vi "FindIP.vi"(2 "error in 2":errorcluster, 3 "String":string) -> (0 "error out":errorcluster, 1 "Numeric":u32)   [LabVIEW 2010]
uses:
  <vilib>/Utility/file.llb/Read From Spreadsheet File (string).vi
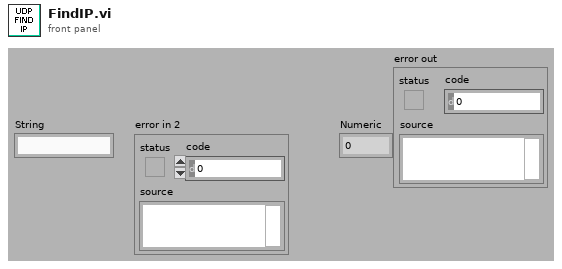
[diagram p1: front panel]
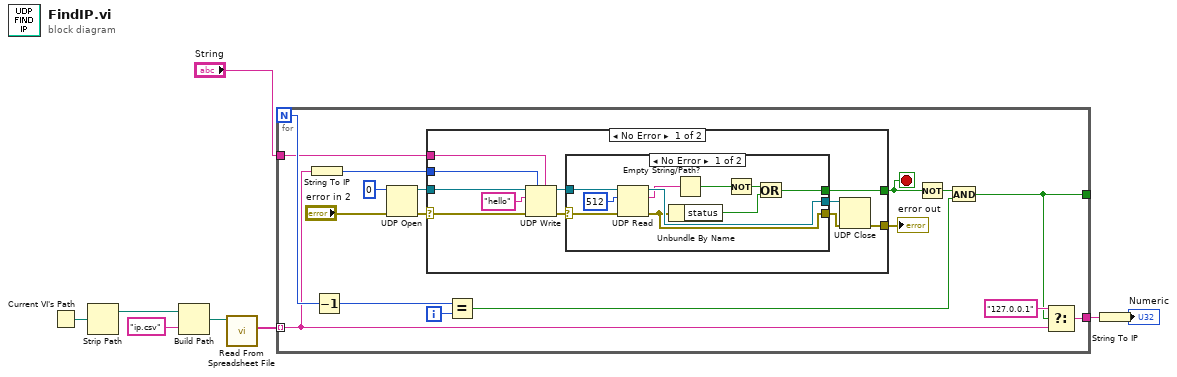
[diagram p0: block diagram]
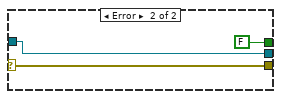
[diagram p2: hidden frame]
diagram:
  n1 = Current VI's Path() -> (path=w2:path)
  n2 = Strip Path(path=w2) -> (stripped path=w3:path)  [unwired: 1 out]
  n3 = Build Path(base path=w3, name or relative path="ip.csv") -> (appended path=w5:path)
  n4 = call-poly <vilib>:"Read From Spreadsheet File.vi"("file path (dialog if empty)"=w5) -> ("first row"=w6:string[])  [unwired: 6 in, 4 out]
  n5 = for {
    N -> [w20]
    tunnel: [w21] -> _
    tunnel: w6 -> [w14] mode=indexing
    tunnel: [w23] -> w7
    tunnel: "String" -> [w12]
    i -> [w25]
    stop <- w11 stop-if-true
    n6 = String To IP(1:w14) -> (0:w13:u32)
    n7 = Decrement(x=w20) -> (x-1=w19:i32)
    n8 = UDP Open(8:"error in 2", 11:u16 0 ("port")) -> (port=w15:refnum<k16>, 0:w16:errorcluster)  [unwired: 3 in, 1 out]
    n9 = case shown="No Error" w16 {
      selector: w16 -> [w36 w50]
      tunnel: [w31 w50] -> w9
      tunnel: w15 -> [w29 _]
      tunnel: [w28 _] -> w11
      tunnel: w13 -> [w27 _]
      tunnel: w12 -> [w26 _]
      frame No Error {
        n10 = UDP Write(address=w27, port or service name=w26, connection ID=w29, data in="hello", 8:w36) -> (error out=w35:errorcluster, 3:w34:refnum<k16>)  [unwired: 1 in]
        n11 = case shown="No Error" w35 {
          selector: w35 -> [w46 w48]
          tunnel: w34 -> [w45 w49]
          tunnel: [w43 w49] -> w33
          tunnel: [w40 w48] -> w32
          tunnel: [w38 FALSE] -> w28
          frame No Error {
            n12 = UDP Read(connection ID=w45, max size (548)=512, 8:w46) -> (data out=w42:string, error out=w40:errorcluster, 3:w43:refnum<k16>)  [unwired: 1 in, 2 out]
            n13 = Unbundle By Name(w40) -> ("status"=w37:bool)
            n14 = Empty String/Path?(string/path=w42) -> (empty?=w41:bool)
            n15 = Not(x=w41) -> (.not. x?=w39:bool)
            n16 = Or(x=w39, y=w37) -> (x .or. y?=w38:bool)
          }
          frame Error {
          }
        }
        n17 = UDP Close(connection ID=w33, 8:w32) -> (error out=w31:errorcluster)  [unwired: 1 out]
      }
      frame Error {
      }
    }
    "error out" <- w9
    n18 = Equal?(x=w19, y=w25) -> (x = y?=w24:bool)
    n19 = Not(x=w11) -> (.not. x?=w10:bool)
    n20 = And(x=w10, y=w24) -> (x .and. y?=w21:bool)
    n21 = Select(t="127.0.0.1", s=w21, f=w14) -> (s? t:f=w23:string)
  }
  n22 = String To IP(1:w7) -> (0:→"Numeric":u32)
